vi "WriteCCWTravelLimit.vi"(8 "error in":errorcluster, 10 "CCWTravelLimit":dbl, 11 "VISA resource name":refnum<visa-resource-name>) -> (0 "error out":errorcluster, 3 "VISA resource name out":refnum<visa-resource-name>)   [LabVIEW 2019, in "Mark 10 TSTM-DC.lvlib"]
uses:
  Mark 10 TSTM-DC.lvlib
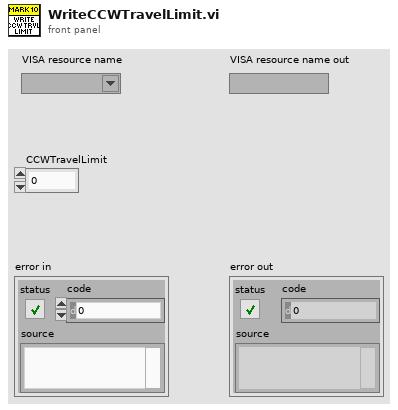
[diagram p1: front panel]
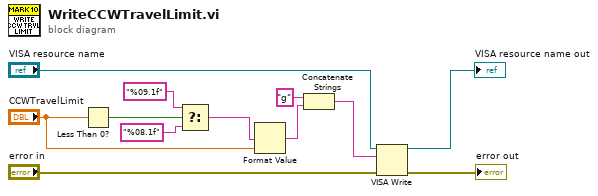
[diagram p0: block diagram]
diagram:
  n1 = Less Than 0?(x="CCWTravelLimit") -> (x < 0?=w4:bool)
  n2 = Select(t="%09.1f" ("format string"), s=w4, f="%08.1f" ("format string")) -> (s? t:f=w1:string)
  n3 = Format Value(format string=w1, value (0)="CCWTravelLimit") -> (output string=w6:string)  [unwired: 1 in]
  n4 = Concatenate Strings("g" ("write buffer"), w6) -> (w7:string)
  n5 = VISA Write(VISA resource name="VISA resource name", write buffer=w7, error in (no error)="error in") -> (VISA resource name out=→"VISA resource name out":refnum<visa-resource-name>, error out=→"error out":errorcluster)  [unwired: 1 out]
